vi "Get Absolute XY.vi"(8 "error in (no error)":errorcluster, 9 "Fiducial?":bool, 10 "input cluster":T1, 11 "Gantry In":refnum<k24>) -> (0 "error out":errorcluster, 2 "Abs XY":dbl[](array[numeric]), 3 "Gantry Out":refnum<k24>)   [LabVIEW 2021, in "Component Tray.lvclass"]
uses:
  Component Tray.lvclass
  C:/Program Files (x86)/Aerotech/A3200/LabVIEW/2010/Bin/Aerotech.A3200.dll
  Program Files (x86)/Aerotech/A3200/LabVIEW/2010/Bin/Aerotech.A3200.dll
  Find Component.ctl
  Controller/Camera/Machine Vision.ctl
  Controller/Motion/A3200/A3200.lvclass
  Controller/Camera/Camera.lvclass
panel:
  out "Error?":bool
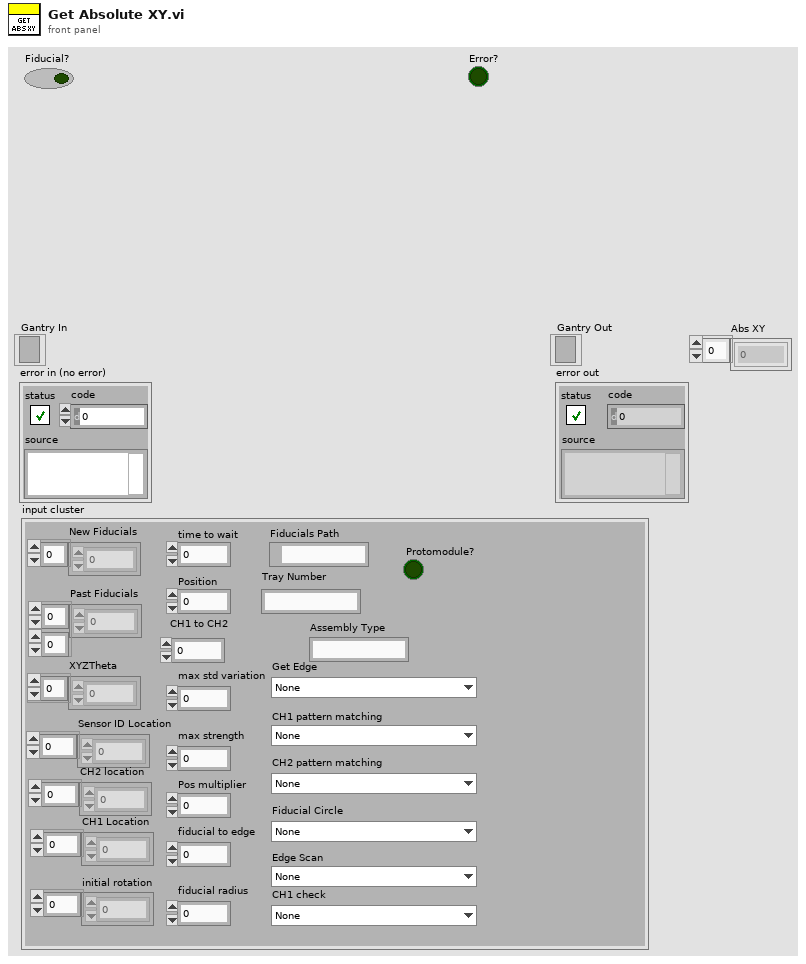
[diagram p1: front panel]
types:
  T1 = typedef "Component Tray.lvclass/Find Component.ctl" = cluster{"New Fiducials":dbl[], "Past Fiducials":dbl[][], "XYZTheta":dbl[], "Fiducials Path":path, "Position":i32, "CH1 Location":dbl[], "Sensor ID Location":dbl[], "initial rotation":dbl[], "CH2 location":dbl[], "max std variation":dbl, "max strength":dbl, "CH2 pattern matching":T2, "Fiducial Circle":T2, "Get Edge":T2, "Pos multiplier":dbl, "time to wait":u32, "fiducial to edge":dbl, "Protomodule?":bool, "Assembly Type":string, "CH1 to CH2":dbl, "Tray Number":string, "fiducial radius":dbl, "4 fiducials?":bool, "CH1 check":T2, "Edge Scan":T2, "CH1 pattern matching":T2, "Sensor Thickness":dbl}
  T2 = typedef "Camera.lvclass/Machine Vision.ctl" = enum16{"None", "Assembly Tray Circle", "Assembly Tray Fiducial", "Partial Hexaboard", "sensor edge init", "HB edge init", "sensor edge pos1", "sensor edge pos2", "HB edge pos1", "HB edge pos2", "Sensor CH1-2", "HB CH1", "HB CH2", "V3 Sensor Circle", "Hexaboard Circle", "sensor CH1 check", "HB CH1 check "}
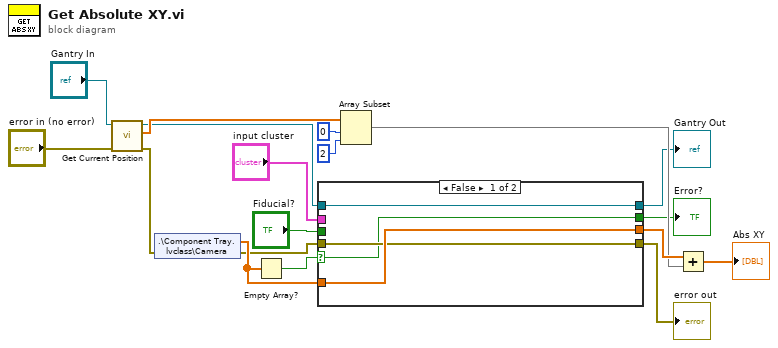
[diagram p0: block diagram]
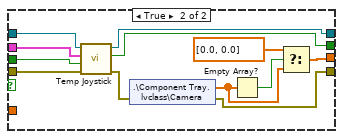
[diagram p2: hidden frame]
diagram:
  n1 = call "Get Current Position.vi"("error in (no error)"="error in (no error)", "Gantry In"="Gantry In") -> ("error out"=w10:errorcluster, "XYZTheta Out"=w14:dbl[], "Gantry Out"=w7:refnum<k24>)  [unwired: 7 in]
  n2 = shared-variable ".\\Component Tray.lvclass\\Camera"(error in=w10) -> (w8:dbl[], error out=w4:errorcluster)
  n3 = Empty Array?(array=w8) -> (empty?=w9:bool)
  n4 = case shown="False" w9 {
    selector: w9 -> [w19 _]
    tunnel: [w22 w23] -> w17
    tunnel: w8 -> [w22 _]
    tunnel: w7 -> [w21 w34]
    tunnel: [w21 w33] -> w6
    tunnel: "input cluster" -> [_ w32]
    tunnel: w4 -> [w20 w31]
    tunnel: [w20 w27] -> w3
    tunnel: "Fiducial?" -> [_ w30]
    tunnel: [w19 w29] -> w1
    frame False {
    }
    frame True {
      n5 = call "Temp Joystick.vi"("error in (no error)"=w31, "Fiducial?"=w30, "Component"=w32, "Gantry In"=w34) -> ("error out"=w28:errorcluster, "Error?"=w29:bool, "Gantry Out"=w33:refnum<k24>)  [unwired: 5 in]
      n6 = shared-variable ".\\Component Tray.lvclass\\Camera"(error in=w28) -> (w26:dbl[], error out=w27:errorcluster)
      n7 = Empty Array?(array=w26) -> (empty?=w25:bool)
      n8 = Select(t=dbl[] [0.0, 0.0], s=w25, f=w26) -> (s? t:f=w23:dbl[])
    }
  }
  "Gantry Out" <- w6
  "error out" <- w3
  "Error?" <- w1
  n9 = Array Subset(array=w14, index=0, length=2) -> (w11:dbl[])
  n10 = Add(x=w17, y=w11) -> (x+y=→"Abs XY":dbl[])
